vi "UNIX Timestamp to LabVIEW Timestamp.vi"(11 "UNIX time stamp":dbl) -> (3 "LabVIEW Timestamp":timestamp)   [LabVIEW 2021, in "Open Weather Session.lvclass"]
uses:
  Open Weather Session.lvclass
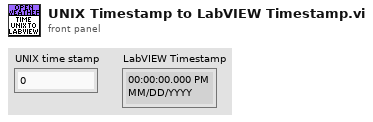
[diagram p1: front panel]
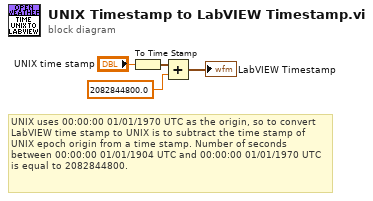
[diagram p0: block diagram]
diagram:
  # "UNIX uses 00:00:00 01/01/1970 UTC as the origin, so to convert LabVIEW time stamp to UNIX is to subtract the time stamp of UNIX epoch origin from a time stamp. Number of seconds between 00:00:00 01/01/1904 UTC and 00:00:00 01/01/1970 UTC is equal to 2082844800."
  n1 = To Time Stamp(1:"UNIX time stamp") -> (0:w2:timestamp)
  n2 = Add(x=w2, y=2082844800.0 ("number")) -> (x+y=→"LabVIEW Timestamp":timestamp)
